vi "main.vi"() -> ()   [LabVIEW 2013]
uses:
  <vilib>/userdefined/High Color/IMAQdx.ctl
  <vilib>/vision/driver/NI_Vision_Acquisition_Software.lvlib
panel:
  out "error out":errorcluster
  out "AVI":path
  in  "stop":bool
  out "image":T1(plugin-control)
  in  "Session In":T2
  in  "Path":path
  in  "File number":i32
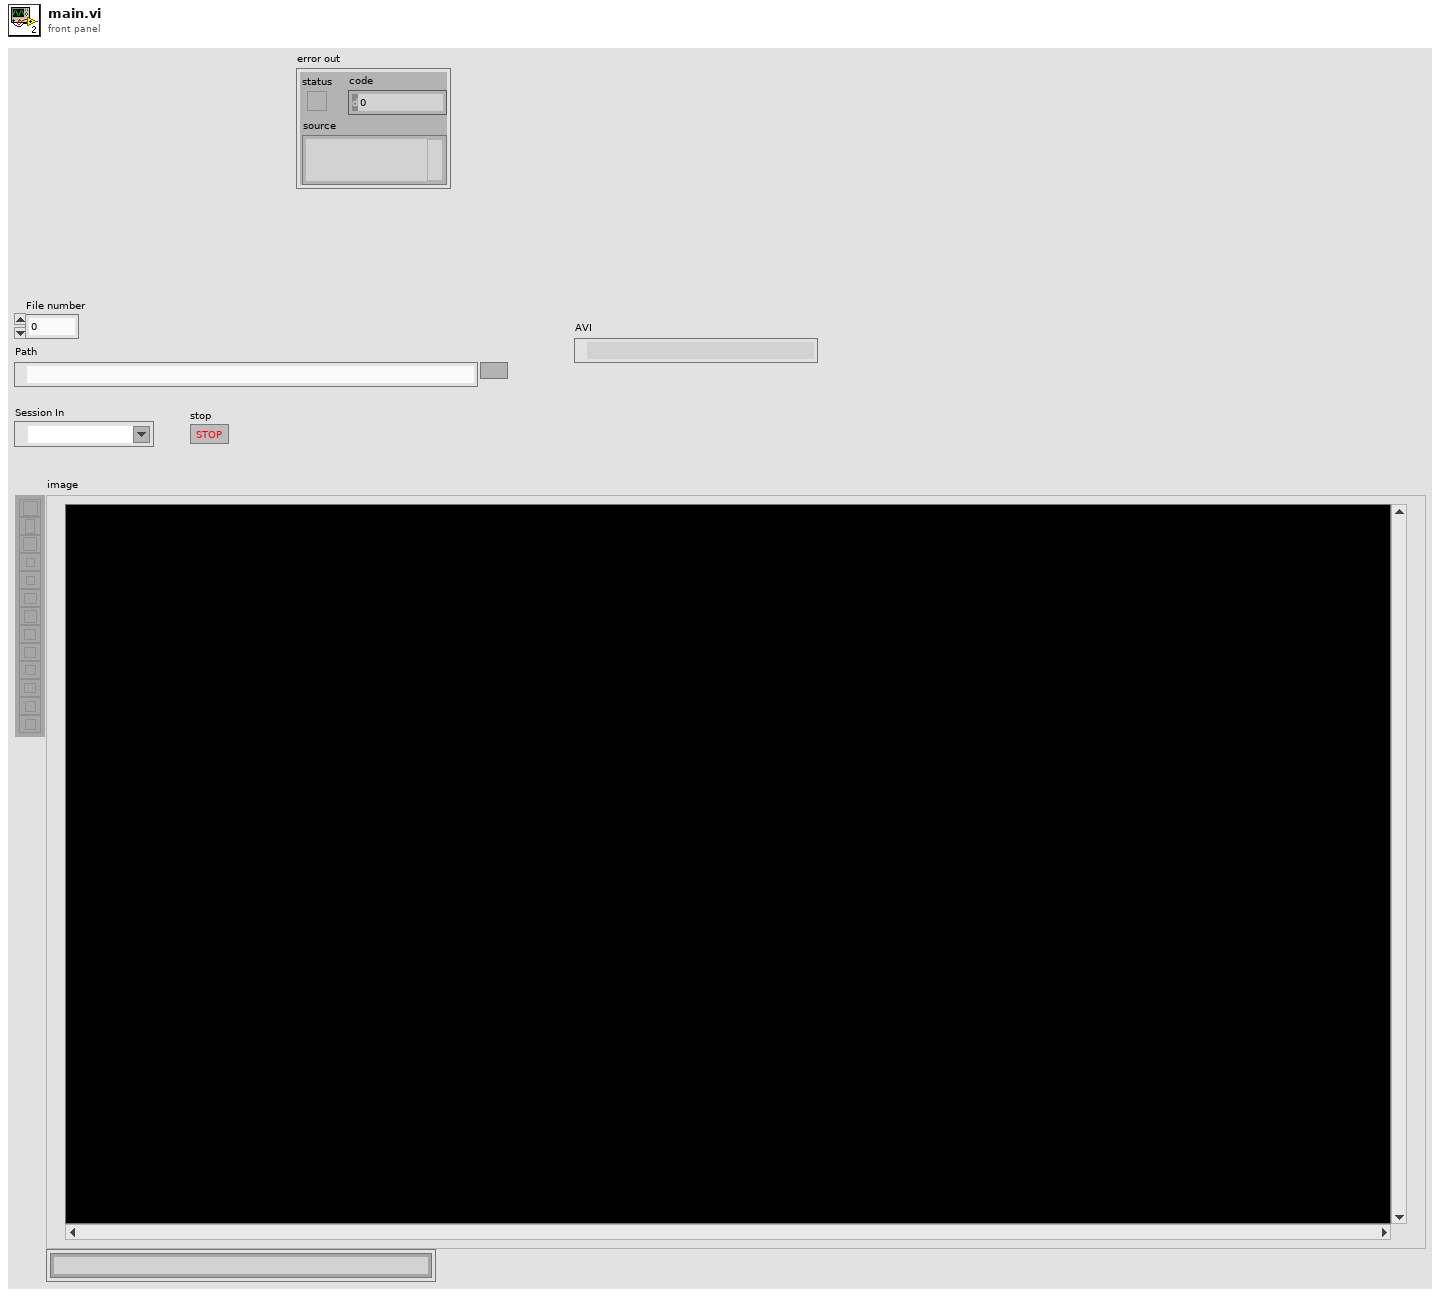
[diagram p1: front panel]
types:
  T1 = typedef "IMAQ Image.ctl" = refnum<image>
  T2 = typedef "IMAQdx.ctl" = refnum<k21>
  T3 = typedef "Image Type" = u32
  T4 = typedef "IMAQ AVI2 Refnum.ctl" = refnum<k20>
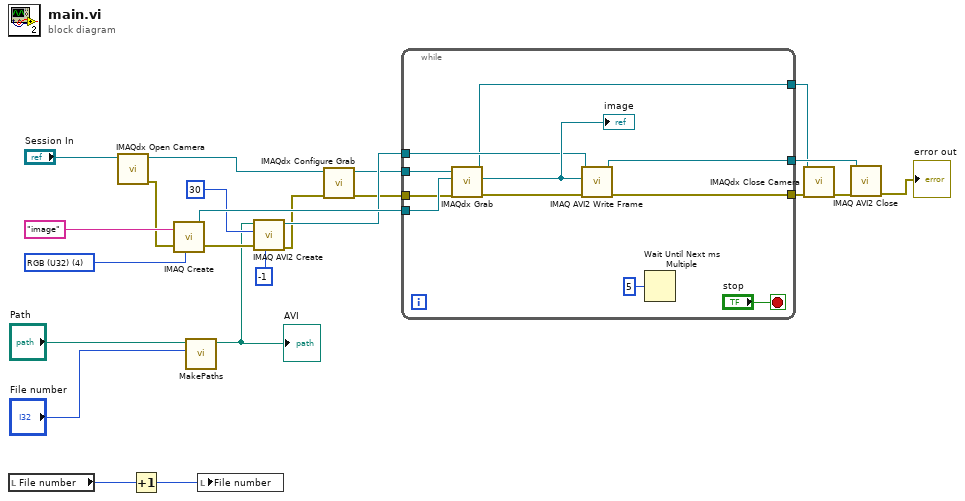
[diagram p0: block diagram]
diagram:
  w18 = T3 4 items=["Grayscale (U8)", "Grayscale (I16)", "Grayscale (SGL)", "Complex (CSG)", "RGB (U32)", "HSL (U32)", "RGB (U64)", "Grayscale (U16)"] ("Image Type")
  n1 = local read "File number"() -> (w2:i32)
  n2 = call <vilib>:"IMAQdx Open Camera.vi"("Session In"="Session In") -> ("error out"=w10:errorcluster, "Session Out"=w5:T2)  [unwired: 9 in]
  n3 = Increment(x=w2) -> (x+1=w1:i32)
  n4 = call "IMAQ Create"("Image Name"="image", "Image Type"=w18, "error in (no error)"=w10) -> ("New Image"=w19:T1, "error out"=w11:errorcluster)  [unwired: 2 in]
  n5 = call "MakePaths.vi"("number"="File number", "Path"="Path") -> ("AVI"=w8:path)  [unwired: 7 in, 2 out]
  "AVI" <- w8
  n6 = local write "File number"(w1) -> ()
  n7 = call "IMAQ AVI2 Create"("Quality"=-1, "error in (no error)"=w11, "Frames Per Second"=u32 30, "AVI Path"=w8) -> ("error out"=w7:errorcluster, "AVI Refnum"=w16:T4)  [unwired: 6 in]
  n8 = call <vilib>:"IMAQdx Configure Grab.vi"("error in"=w7, "Session In"=w5) -> ("error out"=w6:errorcluster, "Session Out"=w4:T2)  [unwired: 8 in]
  n9 = while {
    tunnel: w19 -> [w34]
    tunnel: [w31] -> w17
    tunnel: w16 -> [w29]
    tunnel: [w28] -> w14
    tunnel: [w27] -> w13
    tunnel: w6 -> [w26]
    tunnel: w4 -> [w25]
    stop <- "stop" stop-if-true
    n10 = call <vilib>:"IMAQdx Grab.vi"("error in"=w26, "Image In"=w34, "Session In"=w25) -> ("error out"=w32:errorcluster, "Image Out"=w30:T1, "Session Out"=w27:T2)  [unwired: 5 in, 1 out]
    "image" <- w30
    n11 = call "IMAQ AVI2 Write Frame"("error in (no error)"=w32, "Image"=w30, "AVI Refnum"=w29) -> ("error out"=w31:errorcluster, "AVI Refnum (duplicate)"=w28:T4)  [unwired: 6 in, 1 out]
    n12 = Wait Until Next ms Multiple(millisecond multiple=u32 5) -> ()  [unwired: 1 out]
  }
  n13 = call <vilib>:"IMAQdx Close Camera.vi"("error in"=w17, "Session In"=w13) -> ("error out"=w15:errorcluster)  [unwired: 9 in]
  n14 = call "IMAQ AVI2 Close"("error in (no error)"=w15, "AVI Refnum"=w14) -> ("error out"=→"error out":errorcluster)  [unwired: 9 in]
